vi "Data Socket panel  Writer.vi"() -> ()   [LabVIEW 2012]
doc: "© Copyright M. Ferrari 2012 \n[LV 2009]"
panel:
  in  "stop":bool
  in  "Scale Fact":dbl(knob)=1.0 scale=1.0..10.0
  out "Waveform Chart":dbl(graph)
  # "DATA SOCKET PUBLISHER (WRITER)"
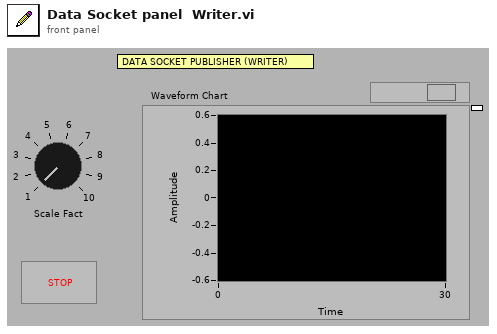
[diagram p1: front panel]
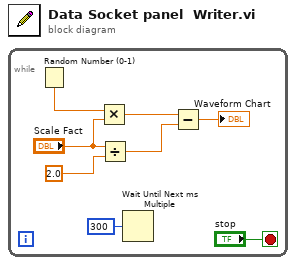
[diagram p0: block diagram]
diagram:
  n1 = while {
    stop <- "stop" stop-if-true
    n2 = Random Number (0-1)() -> (number: 0 to 1=w8:dbl)
    n3 = Multiply(x=w8, y="Scale Fact") -> (x*y=w7:dbl)
    n4 = Divide(x="Scale Fact", y=2.0) -> (x/y=w3:dbl)
    n5 = Wait Until Next ms Multiple(millisecond multiple=u32 300) -> ()  [unwired: 1 out]
    n6 = Subtract(x=w7, y=w3) -> (x-y=→"Waveform Chart":dbl)
  }
